vi "pco.labview_Simple_Example.vi"() -> ()   [LabVIEW 2020]
uses:
  CameraAccess.lvlib
  Structures.lvlib
  Recorder.lvlib
  RecordingControl.lvlib
  TimingControl.lvlib
  GeneralCameraControl.lvlib
panel:
  out "Recorded Images":u32
  out "Image":u16[][](graph)
  in  "Quit":bool
  in  "roiY1":u16=2 min=2 step=1
  in  "roiX1":u16=2 min=2 step=1
  in  "roiY0":u16=1 min=1 step=1
  in  "roiX0":u16=1 min=1 step=1
  out "Image Height":u16
  out "Image Width":u16
  in  "Image Index":u32 max=9
  in  "dwImgCount":u32=10 caption="Required Number of Images" max=4023
  out "Error":errorcluster {"code" format="%x"}
  # "This example shows a simple recording of an image sequence and the image access afterwards.\nIt is a good starting point for writing own applications.\nBut it will not be fail save, i.e. doesnt react on errors, just handles them forward to the end\n\nUsage:\nSelect your required image count before you start the program.\nOnce started, the camera will be opened, the recorder will be created, initialized and images will be recorded automatically.\nWhen acquisition has finished you can address the images and set a certain roi \nTo finish the program click on quit application, this will force free and delete of the recorder and a close camera"
  # "pco.labview"
  # "Camera Setup"
  # "Recording Control"
  # "Parameters for image readout"
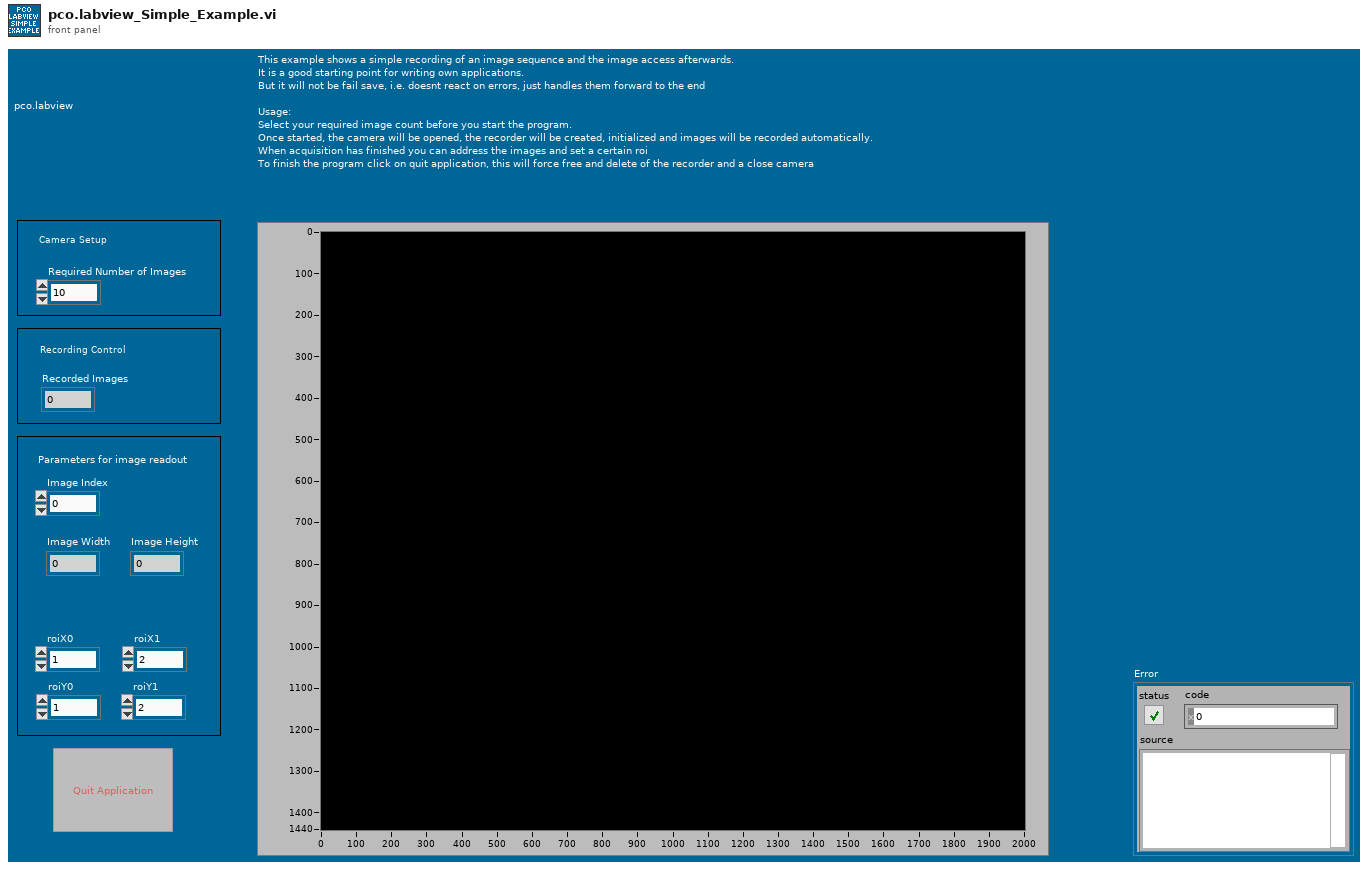
[diagram p1: front panel]
types:
  T1 = enum8{"Enabled", "Disabled", "Disabled and Grayed Out"}
  T2 = cluster{"wInterfaceType":u16, "wCameraNumber":u16, "wCameraNumAtInterface":u16, "wOpenFlags":u16[], "dwOpenFlags":u32[], "wOpenPtr":u64[]}
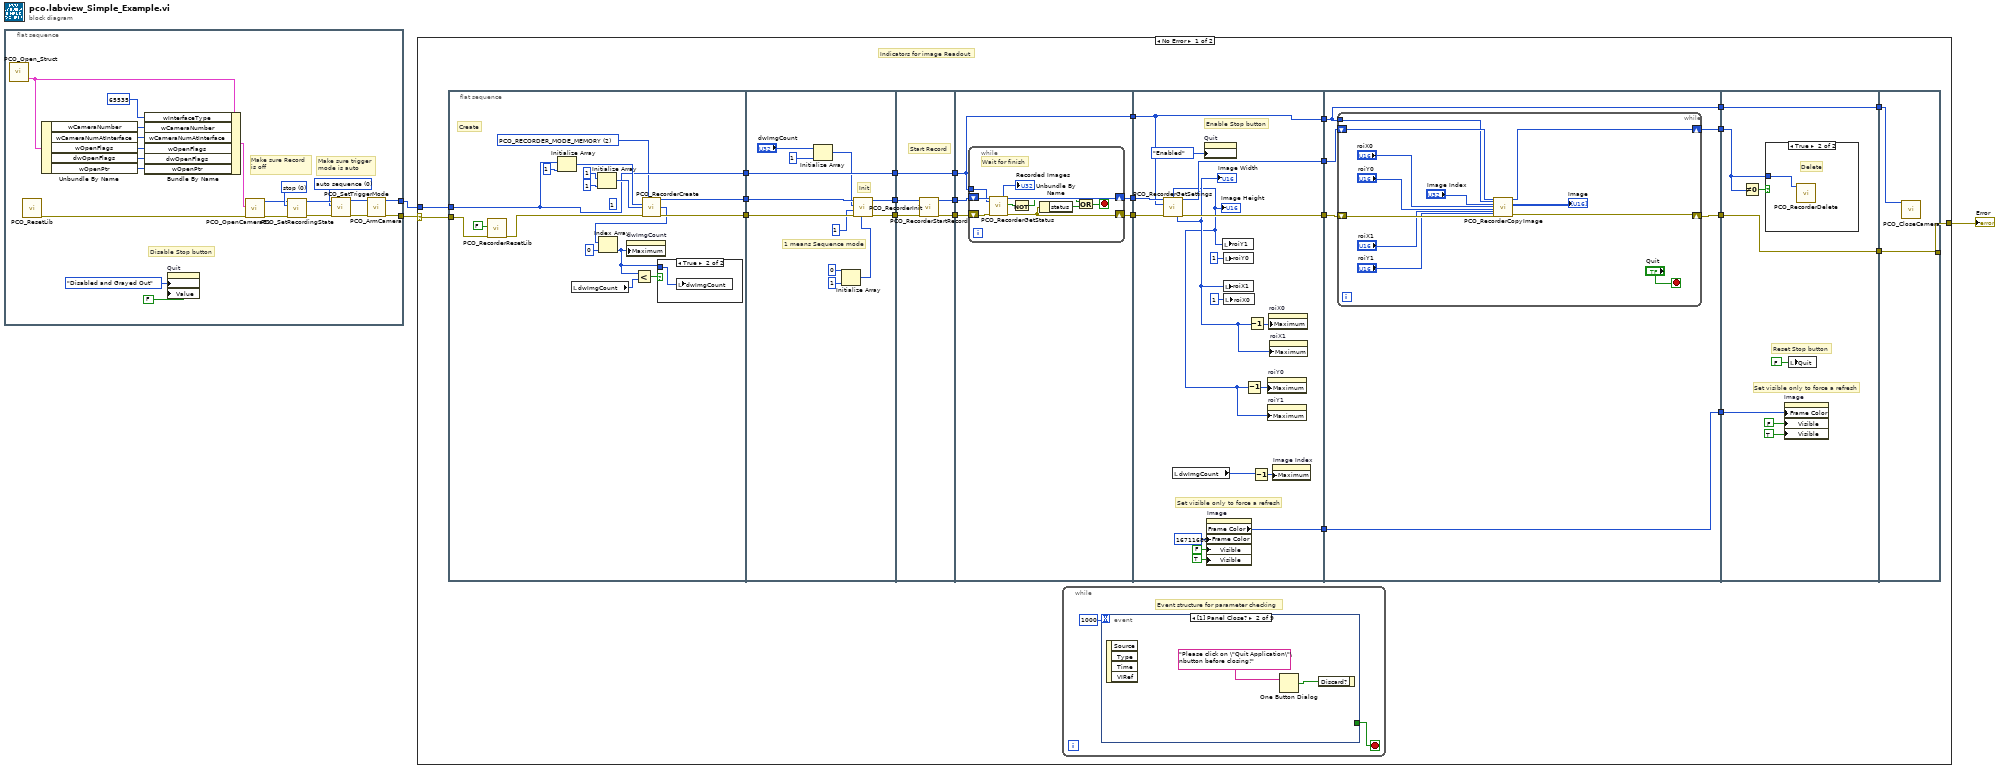
[diagram p0: block diagram]
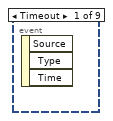
[diagram p2: hidden frame]
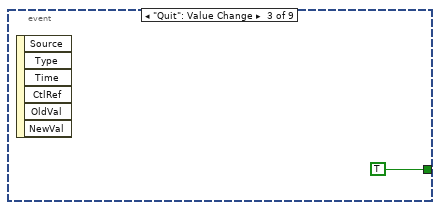
[diagram p3: hidden frame]
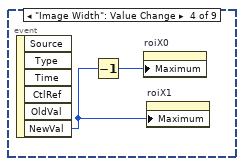
[diagram p4: hidden frame]
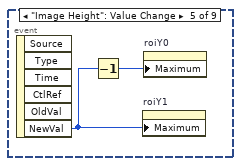
[diagram p5: hidden frame]
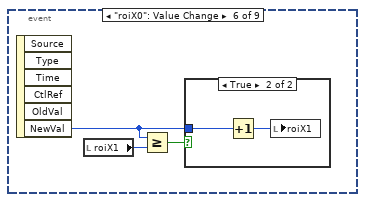
[diagram p6: hidden frame]
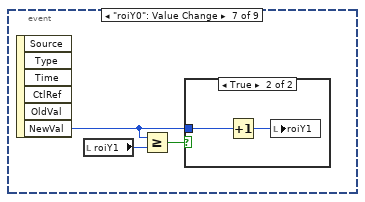
[diagram p8: hidden frame]
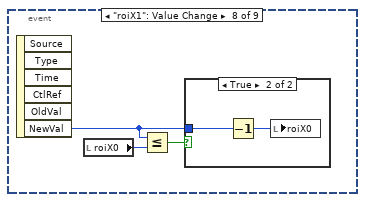
[diagram p10: hidden frame]
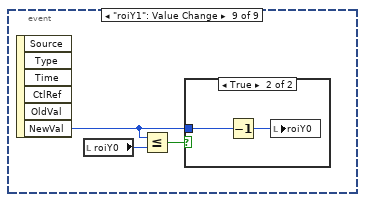
[diagram p12: hidden frame]
diagram:
  n1 = flat-sequence {
    tunnel: [w4] -> w3
    tunnel: [w5] -> w1
    frame #0 {
      w8 = u16 0 items=["auto sequence"=0, "software trigger"=1, "external exposure start & software trigger"=2, "external exposure control"=3, "external synchronized"=4, "fast external exposure control"=5, "external CDS control"=6, "slow external exposure control"=7, "external synchronized HDSDI"=258] ("wTriggerMode")
      w13 = u16 0 items=["stop", "run"] ("wRecState")
      # "Make sure trigger\nmode is auto"
      # "Make sure Record \nis off"
      # "Disable Stop button"
      n2 = call "PCO_Open_Struct.vi"() -> ("PCO_Open_Struct"=w20:T2)  [unwired: 4 in, 4 out]
      n3 = call "PCO_ResetLib.vi"() -> ("error out"=w24:errorcluster)  [unwired: 10 in, 1 out]
      n4 = Unbundle By Name(w20) -> ("wCameraNumber"=w19:u16, "wCameraNumAtInterface"=w18:u16, "wOpenFlags"=w17:u16[], "dwOpenFlags"=w16:u32[], "wOpenPtr"=w15:u64[])
      n5 = Bundle By Name(cluster=w20, "wInterfaceType"=u16 65535, "wCameraNumber"=w19, "wCameraNumAtInterface"=w18, "wOpenFlags"=w17, "dwOpenFlags"=w16, "wOpenPtr"=w15) -> (w14:T2)
      n6 = property on="Quit" class="Bool (strict)"("DisabledEnum"=T1."Disabled and Grayed Out" ("Disabled"), "Value"=FALSE ("Stop")) -> ()  [unwired: 2 in, 2 out]
      n7 = call "PCO_OpenCameraEx.vi"("error in (no error)"=w24, "strOpenStruct"=w14) -> ("error out"=w12:errorcluster, "ph out"=w11:u64)  [unwired: 7 in, 1 out]
      n8 = call "PCO_SetRecordingState.vi"("error in (no error)"=w12, "wRecState"=w13, "ph"=w11) -> ("error out"=w9:errorcluster, "ph out"=w10:u64)  [unwired: 6 in, 1 out]
      n9 = call "PCO_SetTriggerMode.vi"("error in (no error)"=w9, "wTriggerMode"=w8, "ph"=w10) -> ("error out"=w6:errorcluster, "ph out"=w7:u64)  [unwired: 6 in, 1 out]
      n10 = call "PCO_ArmCamera.vi"("error in (no error)"=w6, "ph"=w7) -> ("error out"=w5:errorcluster, "ph out"=w4:u64)  [unwired: 7 in, 1 out]
    }
  }
  n11 = case shown="No Error" w1 {
    selector: w1 -> [w29 w176]
    tunnel: [w25 w176] -> w2
    tunnel: w3 -> [w49 _]
    frame No Error {
      # "Indicators for image Readout"
      n12 = flat-sequence {
        tunnel: w49 -> [w89]
        tunnel: w29 -> [w86]
        tunnel: [w88] -> w48
        tunnel: [w90] -> w47
        tunnel: [w89] -> w36
        tunnel: w48 -> [w108]
        tunnel: w47 -> [w104]
        tunnel: [w107] -> w46
        tunnel: [w106] -> w45
        tunnel: [w105] -> w37
        tunnel: w36 -> [w105]
        tunnel: w46 -> [w113]
        tunnel: w45 -> [w112]
        tunnel: [w111] -> w44
        tunnel: [w110] -> w43
        tunnel: [w109] -> w38
        tunnel: w37 -> [w109]
        tunnel: w44 -> [w118]
        tunnel: w43 -> [w117]
        tunnel: [w116] -> w42
        tunnel: [w115] -> w41
        tunnel: w38 -> [w114]
        tunnel: [w114] -> w35
        tunnel: w42 -> [w145]
        tunnel: w41 -> [w144]
        tunnel: [w143] -> w40
        tunnel: [w142] -> w39
        tunnel: w35 -> [w141]
        tunnel: [w141] -> w34
        tunnel: [w137] -> w28
        tunnel: w40 -> [w152]
        tunnel: w39 -> [w151]
        tunnel: w34 -> [w148]
        tunnel: [w150] -> w33
        tunnel: [w149] -> w32
        tunnel: [w148] -> w31
        tunnel: w28 -> [w147]
        tunnel: [w147] -> w27
        tunnel: w33 -> [w165]
        tunnel: w32 -> [w171]
        tunnel: w31 -> [w169]
        tunnel: [w169] -> w30
        tunnel: w27 -> [w166]
        tunnel: [w165] -> w26
        tunnel: w30 -> [w175]
        tunnel: w26 -> [w174]
        tunnel: [w174] -> w25
        frame #0 {
          w79 = u16 2 items=["PCO_RECORDER_MODE_FILE"=1, "PCO_RECORDER_MODE_MEMORY"=2, "PCO_RECORDER_MODE_CAMRAM"=3] ("dwRecMode")
          (unwired) u16 1 ("wArrLength")
          # "Create"
          n13 = call "PCO_RecorderResetLib.vi"("error in (no error)"=w86, "bSilent"=FALSE) -> ("error out"=w85:errorcluster)  [unwired: 8 in, 1 out]
          n14 = Initialize Array(w89, u32 1 ("element")) -> (w94:u64[])
          n15 = local read "dwImgCount"() -> (w82:u32)
          n16 = Initialize Array(u32 1 ("element"), u32 1 ("element")) -> (w91:u32[])
          n17 = call "PCO_RecorderCreate.vi"("wRecMode"=w79, "phCamArr"=w94, "dwImgDistributionArr"=w91, "error in (no error)"=w85) -> ("phRec out"=w88:u64, "dwMaxImgCountArr"=w84:u32[], "error out"=w90:errorcluster)  [unwired: 8 in, 1 out]
          n18 = Index Array(array=w84, index=0) -> (element=w81:u32)
          n19 = property on="dwImgCount" class="DigNum (strict)"("Maximum"=w81) -> ()  [unwired: 2 in, 2 out]
          n20 = Less?(x=w81, y=w82) -> (x < y?=w80:bool)
          n21 = case shown="True" w80 {
            tunnel: w81 -> [_ w96]
            frame False {
            }
            frame True {
              n22 = local write "dwImgCount"(w96) -> ()
            }
          }
        }
        frame #1 {
          # "1 means Sequence mode"
          # "Init"
          n23 = Initialize Array("dwImgCount", 1 ("dimension size")) -> (w101:u32[])
          n24 = Initialize Array(u16 0 ("element"), 1 ("dimension size")) -> (w97:u16[])
          n25 = call "PCO_RecorderInit.vi"("wRamSegmentArr"=w97, "error in (no error)"=w104, "wType"=u16 1, "dwImgCountArr"=w101, "phRec"=w108) -> ("error out"=w106:errorcluster, "phRec out"=w107:u64)  [unwired: 4 in, 1 out]
        }
        frame #2 {
          # "Start Record"
          n26 = call "PCO_RecorderStartRecord.vi"("error in (no error)"=w112, "phRec"=w113) -> ("error out"=w111:errorcluster, "phRec out"=w110:u64)  [unwired: 7 in, 1 out]
        }
        frame #3 {
          n27 = while {
            shift-right: [w127] -> w115
            shift-left: w118 -> [w128]
            shift-right: [w123] -> w116
            shift-left: w117 -> [w124]
            tunnel: w114 -> [w122]
            stop <- w125 stop-if-true
            # "Wait for finish"
            n28 = call "PCO_RecorderGetStatus.vi"("phRec"=w124, "phCam"=w122, "error in (no error)"=w128) -> ("dwProcImgCount"=→"Recorded Images":u32, "phRec out"=w123:u64, "bIsRunning"=w121:bool, "error out"=w127:errorcluster)  [unwired: 5 in, 8 out]
            n29 = Not(x=w121) -> (.not. x?=w120:bool)
            n30 = Unbundle By Name(w127) -> ("status"=w126:bool)
            n31 = Or(x=w120, y=w126) -> (x .or. y?=w125:bool)
          }
        }
        frame #4 {
          # "Set visible only to force a refresh"
          # "Enable Stop button"
          n32 = call "PCO_RecorderGetSettings.vi"("phRec"=w145, "phCam"=w141, "error in (no error)"=w144) -> ("wHeight"=w130:u16, "phRec out"=w143:u64, "wWidth"=w131:u16, "error out"=w142:errorcluster)  [unwired: 4 in, 5 out]
          "Image Width" <- w131
          "Image Height" <- w130
          n33 = local read "dwImgCount"() -> (w129:u32)
          n34 = property on="Quit" class="Bool (strict)"("DisabledEnum"=T1."Enabled" ("Disabled")) -> ()  [unwired: 2 in, 2 out]
          n35 = property on="Image" class="IntGraph (strict)"("Frame Color"=u32 16711680, "Visible"=FALSE, "Visible"=TRUE) -> ("Frame Color"=w137:u32)  [unwired: 2 in, 2 out]
          n36 = local write "roiY1"(w130) -> ()
          n37 = local write "roiY0"(u16 1 ("roiY0")) -> ()
          n38 = local write "roiX1"(w131) -> ()
          n39 = local write "roiX0"(u16 1 ("roiY0")) -> ()
          n40 = Decrement(x=w130) -> (x-1=w133:u16)
          n41 = Decrement(x=w131) -> (x-1=w134:u16)
          n42 = Decrement(x=w129) -> (x-1=w132:u32)
          n43 = property on="roiY0" class="DigNum (strict)"("Maximum"=w133) -> ()  [unwired: 2 in, 2 out]
          n44 = property on="roiY1" class="DigNum (strict)"("Maximum"=w130) -> ()  [unwired: 2 in, 2 out]
          n45 = property on="roiX0" class="DigNum (strict)"("Maximum"=w134) -> ()  [unwired: 2 in, 2 out]
          n46 = property on="roiX1" class="DigNum (strict)"("Maximum"=w131) -> ()  [unwired: 2 in, 2 out]
          n47 = property on="Image Index" class="DigNum (strict)"("Maximum"=w132) -> ()  [unwired: 2 in, 2 out]
        }
        frame #5 {
          n48 = while {
            tunnel: w148 -> [w161]
            shift-right: [w160] -> w149
            shift-left: w152 -> [w163]
            shift-right: [w159] -> w150
            shift-left: w151 -> [w162]
            stop <- "Quit" stop-if-true
            n49 = call "PCO_RecorderCopyImage.vi"("phRec"=w163, "phCam"=w161, "dwImgIdx"="Image Index", "wRoiX0"="roiX0", "wRoiY0"="roiY0", "wRoiX1"="roiX1", "wRoiY1"="roiY1", "error in (no error)"=w162) -> ("phRec out"=w160:u64, "wImgBuf"=→"Image":u16[][], "error out"=w159:errorcluster)  [unwired: 13 in, 4 out]
          }
        }
        frame #6 {
          # "Set visible only to force a refresh"
          # "Reset Stop button"
          n50 = Not Equal To 0?(x=w171) -> (x != 0?=w170:bool)
          n51 = case shown="True" w170 {
            tunnel: w171 -> [_ w173]
            frame False {
            }
            frame True {
              # "Delete"
              n52 = call "PCO_RecorderDelete.vi"("phRec"=w173) -> ()  [unwired: 9 in, 2 out]
            }
          }
          n53 = property on="Image" class="IntGraph (strict)"("Frame Color"=w166, "Visible"=FALSE, "Visible"=TRUE) -> ()  [unwired: 2 in, 2 out]
          n54 = local write "Quit"(FALSE ("Stop")) -> ()
        }
        frame #7 {
          n55 = call "PCO_CloseCamera.vi"("ph"=w175) -> ()  [unwired: 9 in, 2 out]
        }
      }
      n56 = while {
        stop <- w50 stop-if-true
        # "Event structure for parameter checking"
        n57 = event shown="[1] Panel Close?" {
          selector: _ -> [_ _ _ _ _ _ _ _ _]
          dyn-events: _ -> [_ _ _ _ _ _ _ _ _]
          timeout: 1000 -> [_ _ _ _ _ _ _ _ _]
          tunnel: [_ _ TRUE _ _ _ _ _ _] -> w50
          event Timeout {
            n58 = event-data() -> ()  [unwired: 1 in, 3 out]
          }
          event Panel Close? {
            n59 = event-data() -> ()  [unwired: 1 in, 4 out]
            n60 = One Button Dialog(message="Please click on \"Quit Application\"\nbutton before closing!") -> (true=w52:bool)  [unwired: 1 in]
            n61 = event-data("Discard?"=w52) -> ()  [unwired: 1 in, 1 out]
          }
          event "Quit": Value Change {
            n62 = event-data() -> ()  [unwired: 1 in, 6 out]
          }
          event "Image Width": Value Change {
            n63 = event-data() -> ("NewVal"=w55:u16)  [unwired: 1 in, 5 out]
            n64 = Decrement(x=w55) -> (x-1=w56:u16)
            n65 = property on="roiX0" class="DigNum (strict)"("Maximum"=w56) -> ()  [unwired: 2 in, 2 out]
            n66 = property on="roiX1" class="DigNum (strict)"("Maximum"=w55) -> ()  [unwired: 2 in, 2 out]
          }
          event "Image Height": Value Change {
            n67 = event-data() -> ("NewVal"=w57:u16)  [unwired: 1 in, 5 out]
            n68 = Decrement(x=w57) -> (x-1=w58:u16)
            n69 = property on="roiY1" class="DigNum (strict)"("Maximum"=w57) -> ()  [unwired: 2 in, 2 out]
            n70 = property on="roiY0" class="DigNum (strict)"("Maximum"=w58) -> ()  [unwired: 2 in, 2 out]
          }
          event "roiX0": Value Change {
            n71 = event-data() -> ("NewVal"=w59:u16)  [unwired: 1 in, 5 out]
            n72 = local read "roiX1"() -> (w61:u16)
            n73 = Greater Or Equal?(x=w59, y=w61) -> (x >= y?=w60:bool)
            n74 = case shown="True" w60 {
              tunnel: w59 -> [_ w63]
              frame False {
              }
              frame True {
                n75 = Increment(x=w63) -> (x+1=w62:u16)
                n76 = local write "roiX1"(w62) -> ()
              }
            }
          }
          event "roiY0": Value Change {
            n77 = event-data() -> ("NewVal"=w64:u16)  [unwired: 1 in, 5 out]
            n78 = local read "roiY1"() -> (w66:u16)
            n79 = Greater Or Equal?(x=w64, y=w66) -> (x >= y?=w65:bool)
            n80 = case shown="True" w65 {
              tunnel: w64 -> [_ w68]
              frame False {
              }
              frame True {
                n81 = Increment(x=w68) -> (x+1=w67:u16)
                n82 = local write "roiY1"(w67) -> ()
              }
            }
          }
          event "roiX1": Value Change {
            n83 = event-data() -> ("NewVal"=w69:u16)  [unwired: 1 in, 5 out]
            n84 = local read "roiX0"() -> (w71:u16)
            n85 = Less Or Equal?(x=w69, y=w71) -> (x <= y?=w70:bool)
            n86 = case shown="True" w70 {
              tunnel: w69 -> [_ w73]
              frame False {
              }
              frame True {
                n87 = Decrement(x=w73) -> (x-1=w72:u16)
                n88 = local write "roiX0"(w72) -> ()
              }
            }
          }
          event "roiY1": Value Change {
            n89 = event-data() -> ("NewVal"=w74:u16)  [unwired: 1 in, 5 out]
            n90 = local read "roiY0"() -> (w76:u16)
            n91 = Less Or Equal?(x=w74, y=w76) -> (x <= y?=w75:bool)
            n92 = case shown="True" w75 {
              tunnel: w74 -> [_ w78]
              frame False {
              }
              frame True {
                n93 = Decrement(x=w78) -> (x-1=w77:u16)
                n94 = local write "roiY0"(w77) -> ()
              }
            }
          }
        }
      }
    }
    frame Error {
    }
  }
  "Error" <- w2
